vi "create.vi"(8 "error in (no error)":errorcluster, 10 "SubnetSettings":T1, 11 "SubnetFactory in":refnum<class "SubnetFactory.lvclass">) -> (0 "error out":errorcluster, 2 "Subnet":refnum<class "Subnet.lvclass">, 3 "SubnetFactory out":refnum<class "SubnetFactory.lvclass">)   [LabVIEW 2016, in "SubnetFactory.lvclass"]
uses:
  SubnetFactory.lvclass
  Subnet/DataTypes/SubnetSettings.ctl
  Common_RT_Modbus/IModbusFactory/IModbusFactory.lvclass
  Common_RT_HPILC/DataTypes/HPSettings.ctl
  Common_RT_ILC/DataTypes/ILCSettings.ctl
  Common_RT_MTILC/DataTypes/MTSettings.ctl
  Common_RT_MDILC/DataTypes/MDSettings.ctl
  Common_RT_MIILC/DataTypes/MISettings.ctl
  Subnet/Subnet.lvclass
  Common_RT_HPILC/HPILCFactory/HPILCFactory.lvclass
  Subnet/DataTypes/SubnetConstants.ctl
  Common_RT_Modbus/IModbus/IModbus.lvclass
  Common_RT_HPILC/HPILC/HPILC.lvclass
  Subnet/DataTypes/ILCIndexData.ctl
  Subnet/DataTypes/ILCTypes.ctl
  Common_RT_MTILC/MTILC/MTILC.lvclass
  Common_RT_MDILC/MDILC/MDILC.lvclass
  Common_RT_MIILC/MIILC/MIILC.lvclass
  Subnet/DataTypes/SubnetData.ctl
  Subnet/DataTypes/SubnetCommand.ctl
  Subnet/DataTypes/SubnetTelemetry.ctl
  Common_RT_MTILC/MTILCFactory/MTILCFactory.lvclass
  Common_RT_MDILC/MDILCFactory/MDILCFactory.lvclass
  Common_RT_MIILC/MIILCFactory/MIILCFactory.lvclass
  Common_RT_ILC/DataTypes/ILCTimings.ctl
  Common_RT_HPILC/DataTypes/HPTimings.ctl
  Common_RT_MTILC/DataTypes/MTTimings.ctl
  Common_RT_MDILC/DataTypes/MDTimings.ctl
  Common_RT_MIILC/DataTypes/MITimings.ctl
  Subnet/Subnet.lvclass/Subnet.ctl
  Common_RT_ILC/RTILC.lvlib
  Common_RT_HPILC/RTHPILC.lvlib
  Common_RT_MTILC/RTMTILC.lvlib
  Common_RT_MDILC/RTMDILC.lvlib
  Common_RT_MIILC/RTMIILC.lvlib
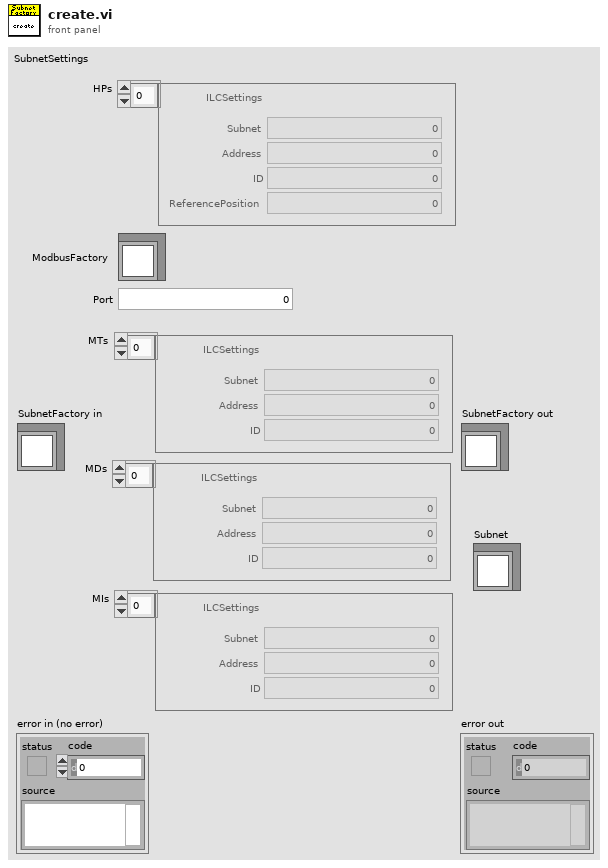
[diagram p1: front panel]
types:
  T1 = typedef "SubnetSettings.ctl" = cluster{"HPs":T2[], "ModbusFactory":refnum<class "IModbusFactory.lvclass">, "Port":i32, "MTs":T4[], "MDs":T5[], "MIs":T6[]}
  T2 = typedef "RTHPILC.lvlib/HPSettings.ctl" = cluster{"ILCSettings":T3, "ID":i16, "ReferencePosition":i32}
  T3 = typedef "RTILC.lvlib/ILCSettings.ctl" = cluster{"Subnet":u8, "Address":u8}
  T4 = typedef "RTMTILC.lvlib/MTSettings.ctl" = cluster{"ILCSettings":T3, "ID":i16}
  T5 = typedef "RTMDILC.lvlib/MDSettings.ctl" = cluster{"ILCSettings":T3, "ID":i16}
  T6 = typedef "RTMIILC.lvlib/MISettings.ctl" = cluster{"ILCSettings":T3, "ID":i16}
  T7 = typedef "RTMIILC.lvlib/MITimings.ctl" = cluster{"Inclination":u32}
  T8 = typedef "RTMDILC.lvlib/MDTimings.ctl" = cluster{"Displacement":u32}
  T9 = typedef "RTMTILC.lvlib/MTTimings.ctl" = cluster{"Temperature":u32}
  T10 = typedef "RTHPILC.lvlib/HPTimings.ctl" = cluster{"BroadcastStepMotor":u32, "ForceAndStatus":u32, "FreezeSensorValues":u32, "StepMotor":u32}
  T11 = typedef "RTILC.lvlib/ILCTimings.ctl" = cluster{"ADCOffsetSensitivity":u32, "ADCScanRate":u32, "ILCMode":u32, "ReadCalibration":u32, "ReportServerID":u32, "ReportServerStatus":u32, "Reset":u32, "SetTemporaryAddress":u32}
  T12 = typedef "SubnetData.ctl" = cluster{"SubnetConstants":T13, "SubnetCommand":T16, "SubnetTelemetry":T17}
  T13 = typedef "SubnetConstants.ctl" = cluster{"Modbus":refnum<class "IModbus.lvclass">, "HPs":refnum<class "HPILC.lvclass">[], "AddressToActuator":T14[], "MTs":refnum<class "MTILC.lvclass">[], "MDs":refnum<class "MDILC.lvclass">[], "MIs":refnum<class "MIILC.lvclass">[]}
  T14 = typedef "ILCIndexData.ctl" = cluster{"ILCTypes":T15, "Index":i32}
  T15 = typedef "ILCTypes.ctl" = enum16{"Undefined", "SAA", "DAA", "HP", "MT", "MD", "MI"}
  T16 = typedef "SubnetCommand.ctl" = cluster{"BroadcastCounter":u8}
  T17 = typedef "SubnetTelemetry.ctl" = cluster{"BytesTransmitted":u32, "FramesTransmitted":u32, "BytesReceived":u32, "FramesReceived":u32, "TxInternalFIFOOverflow":bool, "InvalidInstruction":bool, "WaitForRxFrameTimeout":bool, "StartBitError":bool, "StopBitError":bool, "RxDataFIFOOverflow":bool}
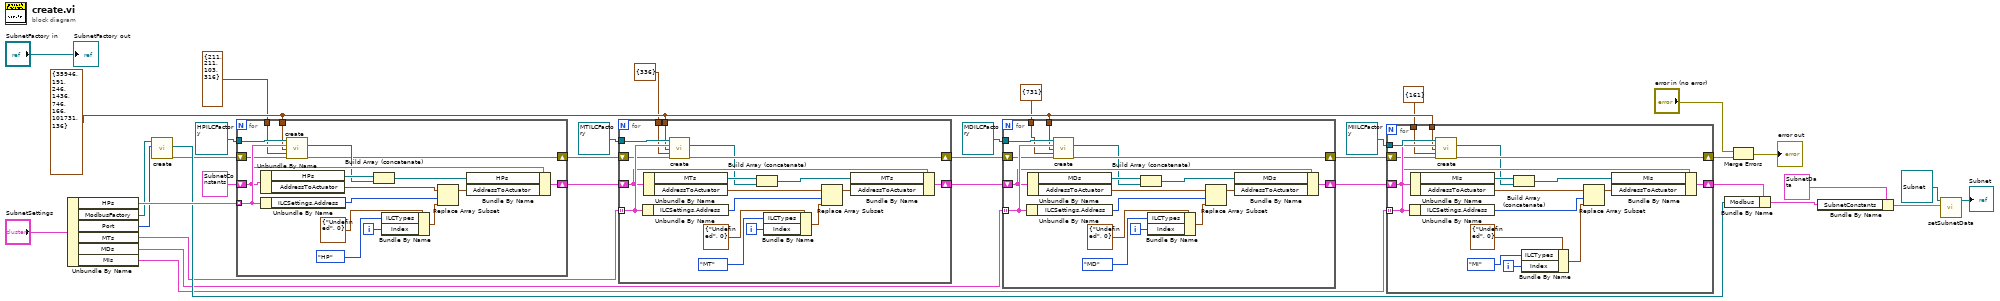
[diagram p0: block diagram]
diagram:
  w5 = T11 {"ADCOffsetSensitivity"=35946, "ADCScanRate"=191, "ILCMode"=246, "ReadCalibration"=1436, "ReportServerID"=746, "ReportServerStatus"=166, "Reset"=101731, "SetTemporaryAddress"=136} ("ILCTimings")
  n1 = Unbundle By Name("SubnetSettings") -> ("HPs"=w33:T2[], "ModbusFactory"=w24:refnum<class "IModbusFactory.lvclass">, "Port"=w23:i32, "MTs"=w19:T4[], "MDs"=w13:T5[], "MIs"=w9:T6[])
  n2 = call-dynamic "create.vi"("Port"=w23, "IModbusFactory in"=w24) -> ("error out"=w21:errorcluster, "IModbus"=w22:refnum<class "IModbus.lvclass">)  [unwired: 7 in, 1 out]
  n3 = for {
    tunnel: w33 -> [w52] mode=indexing
    tunnel: refnum<class "HPILCFactory.lvclass"> refnum ("RTHPILC.lvlib:HPILCFactory.lvclass") -> [w53]
    shift-right: [w43] -> w18
    shift-left: T13 {"Modbus"=refnum, "HPs"=[], "AddressToActuator"=[{"ILCTypes"=enum."Undefined", "Index"=0}, {"ILCTypes"=enum."Undefined", "Index"=0}, {"ILCTypes"=enum."Undefined", "Index"=0}, {"ILCTypes"=enum."Undefined", "Index"=0}, {"ILCTypes"=enum."Undefined", "Index"=0}, {"ILCTypes"=enum."Undefined", "Index"=0}, {"ILCTypes"=enum."Undefined", "Index"=0}, {"ILCTypes"=enum."Undefined", "Index"=0}, {"ILCTypes"=enum."Undefined", "Index"=0}, {"ILCTypes"=enum."Undefined", "Index"=0}, {"ILCTypes"=enum."Undefined", "Index"=0}, {"ILCTypes"=enum."Undefined", "Index"=0}, {"ILCTypes"=enum."Undefined", "Index"=0}, {"ILCTypes"=enum."Undefined", "Index"=0}, {"ILCTypes"=enum."Undefined", "Index"=0}, {"ILCTypes"=enum."Undefined", "Index"=0}, {"ILCTypes"=enum."Undefined", "Index"=0}, {"ILCTypes"=enum."Undefined", "Index"=0}, {"ILCTypes"=enum."Undefined", "Index"=0}, {"ILCTypes"=enum."Undefined", "Index"=0}, {"ILCTypes"=enum."Undefined", "Index"=0}, {"ILCTypes"=enum."Undefined", "Index"=0}, {"ILCTypes"=enum."Undefined", "Index"=0}, {"ILCTypes"=enum."Undefined", "Index"=0}, {"ILCTypes"=enum."Undefined", "Index"=0}, {"ILCTypes"=enum."Undefined", "Index"=0}, {"ILCTypes"=enum."Undefined", "Index"=0}, {"ILCTypes"=enum."Undefined", "Index"=0}, {"ILCTypes"=enum."Undefined", "Index"=0}, {"ILCTypes"=enum."Undefined", "Index"=0}, {"ILCTypes"=enum."Undefined", "Index"=0}, {"ILCTypes"=enum."Undefined", "Index"=0}, {"ILCTypes"=enum."Undefined", "Index"=0}, {"ILCTypes"=enum."Undefined", "Index"=0}, {"ILCTypes"=enum."Undefined", "Index"=0}, {"ILCTypes"=enum."Undefined", "Index"=0}, {"ILCTypes"=enum."Undefined", "Index"=0}, {"ILCTypes"=enum."Undefined", "Index"=0}, {"ILCTypes"=enum."Undefined", "Index"=0}, {"ILCTypes"=enum."Undefined", "Index"=0}, {"ILCTypes"=enum."Undefined", "Index"=0}, {"ILCTypes"=enum."Undefined", "Index"=0}, {"ILCTypes"=enum."Undefined", "Index"=0}, {"ILCTypes"=enum."Undefined", "Index"=0}, {"ILCTypes"=enum."Undefined", "Index"=0}, {"ILCTypes"=enum."Undefined", "Index"=0}, {"ILCTypes"=enum."Undefined", "Index"=0}, {"ILCTypes"=enum."Undefined", "Index"=0}, {"ILCTypes"=enum."Undefined", "Index"=0}, {"ILCTypes"=enum."Undefined", "Index"=0}, {"ILCTypes"=enum."Undefined", "Index"=0}, {"ILCTypes"=enum."Undefined", "Index"=0}, {"ILCTypes"=enum."Undefined", "Index"=0}, {"ILCTypes"=enum."Undefined", "Index"=0}, {"ILCTypes"=enum."Undefined", "Index"=0}, {"ILCTypes"=enum."Undefined", "Index"=0}, {"ILCTypes"=enum."Undefined", "Index"=0}, {"ILCTypes"=enum."Undefined", "Index"=0}, {"ILCTypes"=enum."Undefined", "Index"=0}, {"ILCTypes"=enum."Undefined", "Index"=0}, {"ILCTypes"=enum."Undefined", "Index"=0}, {"ILCTypes"=enum."Undefined", "Index"=0}, {"ILCTypes"=enum."Undefined", "Index"=0}, {"ILCTypes"=enum."Undefined", "Index"=0}, {"ILCTypes"=enum."Undefined", "Index"=0}, {"ILCTypes"=enum."Undefined", "Index"=0}, {"ILCTypes"=enum."Undefined", "Index"=0}, {"ILCTypes"=enum."Undefined", "Index"=0}, {"ILCTypes"=enum."Undefined", "Index"=0}, {"ILCTypes"=enum."Undefined", "Index"=0}, {"ILCTypes"=enum."Undefined", "Index"=0}, {"ILCTypes"=enum."Undefined", "Index"=0}, {"ILCTypes"=enum."Undefined", "Index"=0}, {"ILCTypes"=enum."Undefined", "Index"=0}, {"ILCTypes"=enum."Undefined", "Index"=0}, {"ILCTypes"=enum."Undefined", "Index"=0}, {"ILCTypes"=enum."Undefined", "Index"=0}, {"ILCTypes"=enum."Undefined", "Index"=0}, {"ILCTypes"=enum."Undefined", "Index"=0}, {"ILCTypes"=enum."Undefined", "Index"=0}, {"ILCTypes"=enum."Undefined", "Index"=0}, {"ILCTypes"=enum."Undefined", "Index"=0}, {"ILCTypes"=enum."Undefined", "Index"=0}, {"ILCTypes"=enum."Undefined", "Index"=0}, {"ILCTypes"=enum."Undefined", "Index"=0}, {"ILCTypes"=enum."Undefined", "Index"=0}, {"ILCTypes"=enum."Undefined", "Index"=0}, {"ILCTypes"=enum."Undefined", "Index"=0}, {"ILCTypes"=enum."Undefined", "Index"=0}, {"ILCTypes"=enum."Undefined", "Index"=0}, {"ILCTypes"=enum."Undefined", "Index"=0}, {"ILCTypes"=enum."Undefined", "Index"=0}, {"ILCTypes"=enum."Undefined", "Index"=0}, {"ILCTypes"=enum."Undefined", "Index"=0}, {"ILCTypes"=enum."Undefined", "Index"=0}, {"ILCTypes"=enum."Undefined", "Index"=0}, {"ILCTypes"=enum."Undefined", "Index"=0}, {"ILCTypes"=enum."Undefined", "Index"=0}, {"ILCTypes"=enum."Undefined", "Index"=0}, {"ILCTypes"=enum."Undefined", "Index"=0}, {"ILCTypes"=enum."Undefined", "Index"=0}, {"ILCTypes"=enum."Undefined", "Index"=0}, {"ILCTypes"=enum."Undefined", "Index"=0}, {"ILCTypes"=enum."Undefined", "Index"=0}, {"ILCTypes"=enum."Undefined", "Index"=0}, {"ILCTypes"=enum."Undefined", "Index"=0}, {"ILCTypes"=enum."Undefined", "Index"=0}, {"ILCTypes"=enum."Undefined", "Index"=0}, {"ILCTypes"=enum."Undefined", "Index"=0}, {"ILCTypes"=enum."Undefined", "Index"=0}, {"ILCTypes"=enum."Undefined", "Index"=0}, {"ILCTypes"=enum."Undefined", "Index"=0}, {"ILCTypes"=enum."Undefined", "Index"=0}, {"ILCTypes"=enum."Undefined", "Index"=0}, {"ILCTypes"=enum."Undefined", "Index"=0}, {"ILCTypes"=enum."Undefined", "Index"=0}, {"ILCTypes"=enum."Undefined", "Index"=0}, {"ILCTypes"=enum."Undefined", "Index"=0}, {"ILCTypes"=enum."Undefined", "Index"=0}, {"ILCTypes"=enum."Undefined", "Index"=0}, {"ILCTypes"=enum."Undefined", "Index"=0}, {"ILCTypes"=enum."Undefined", "Index"=0}, {"ILCTypes"=enum."Undefined", "Index"=0}, {"ILCTypes"=enum."Undefined", "Index"=0}, {"ILCTypes"=enum."Undefined", "Index"=0}, {"ILCTypes"=enum."Undefined", "Index"=0}, {"ILCTypes"=enum."Undefined", "Index"=0}, {"ILCTypes"=enum."Undefined", "Index"=0}, {"ILCTypes"=enum."Undefined", "Index"=0}, {"ILCTypes"=enum."Undefined", "Index"=0}, {"ILCTypes"=enum."Undefined", "Index"=0}, {"ILCTypes"=enum."Undefined", "Index"=0}, {"ILCTypes"=enum."Undefined", "Index"=0}, {"ILCTypes"=enum."Undefined", "Index"=0}, {"ILCTypes"=enum."Undefined", "Index"=0}, {"ILCTypes"=enum."Undefined", "Index"=0}, {"ILCTypes"=enum."Undefined", "Index"=0}, {"ILCTypes"=enum."Undefined", "Index"=0}, {"ILCTypes"=enum."Undefined", "Index"=0}, {"ILCTypes"=enum."Undefined", "Index"=0}, {"ILCTypes"=enum."Undefined", "Index"=0}, {"ILCTypes"=enum."Undefined", "Index"=0}, {"ILCTypes"=enum."Undefined", "Index"=0}, {"ILCTypes"=enum."Undefined", "Index"=0}, {"ILCTypes"=enum."Undefined", "Index"=0}, {"ILCTypes"=enum."Undefined", "Index"=0}, {"ILCTypes"=enum."Undefined", "Index"=0}, {"ILCTypes"=enum."Undefined", "Index"=0}, {"ILCTypes"=enum."Undefined", "Index"=0}, {"ILCTypes"=enum."Undefined", "Index"=0}, {"ILCTypes"=enum."Undefined", "Index"=0}, {"ILCTypes"=enum."Undefined", "Index"=0}, {"ILCTypes"=enum."Undefined", "Index"=0}, {"ILCTypes"=enum."Undefined", "Index"=0}, {"ILCTypes"=enum."Undefined", "Index"=0}, {"ILCTypes"=enum."Undefined", "Index"=0}, {"ILCTypes"=enum."Undefined", "Index"=0}, {"ILCTypes"=enum."Undefined", "Index"=0}, {"ILCTypes"=enum."Undefined", "Index"=0}, {"ILCTypes"=enum."Undefined", "Index"=0}, {"ILCTypes"=enum."Undefined", "Index"=0}, {"ILCTypes"=enum."Undefined", "Index"=0}, {"ILCTypes"=enum."Undefined", "Index"=0}, {"ILCTypes"=enum."Undefined", "Index"=0}, {"ILCTypes"=enum."Undefined", "Index"=0}, {"ILCTypes"=enum."Undefined", "Index"=0}, {"ILCTypes"=enum."Undefined", "Index"=0}, {"ILCTypes"=enum."Undefined", "Index"=0}, {"ILCTypes"=enum."Undefined", "Index"=0}, {"ILCTypes"=enum."Undefined", "Index"=0}, {"ILCTypes"=enum."Undefined", "Index"=0}, {"ILCTypes"=enum."Undefined", "Index"=0}, {"ILCTypes"=enum."Undefined", "Index"=0}, {"ILCTypes"=enum."Undefined", "Index"=0}, {"ILCTypes"=enum."Undefined", "Index"=0}, {"ILCTypes"=enum."Undefined", "Index"=0}, {"ILCTypes"=enum."Undefined", "Index"=0}, {"ILCTypes"=enum."Undefined", "Index"=0}, {"ILCTypes"=enum."Undefined", "Index"=0}, {"ILCTypes"=enum."Undefined", "Index"=0}, {"ILCTypes"=enum."Undefined", "Index"=0}, {"ILCTypes"=enum."Undefined", "Index"=0}, {"ILCTypes"=enum."Undefined", "Index"=0}, {"ILCTypes"=enum."Undefined", "Index"=0}, {"ILCTypes"=enum."Undefined", "Index"=0}, {"ILCTypes"=enum."Undefined", "Index"=0}, {"ILCTypes"=enum."Undefined", "Index"=0}, {"ILCTypes"=enum."Undefined", "Index"=0}, {"ILCTypes"=enum."Undefined", "Index"=0}, {"ILCTypes"=enum."Undefined", "Index"=0}, {"ILCTypes"=enum."Undefined", "Index"=0}, {"ILCTypes"=enum."Undefined", "Index"=0}, {"ILCTypes"=enum."Undefined", "Index"=0}, {"ILCTypes"=enum."Undefined", "Index"=0}, {"ILCTypes"=enum."Undefined", "Index"=0}, {"ILCTypes"=enum."Undefined", "Index"=0}, {"ILCTypes"=enum."Undefined", "Index"=0}, {"ILCTypes"=enum."Undefined", "Index"=0}, {"ILCTypes"=enum."Undefined", "Index"=0}, {"ILCTypes"=enum."Undefined", "Index"=0}, {"ILCTypes"=enum."Undefined", "Index"=0}, {"ILCTypes"=enum."Undefined", "Index"=0}, {"ILCTypes"=enum."Undefined", "Index"=0}, {"ILCTypes"=enum."Undefined", "Index"=0}, {"ILCTypes"=enum."Undefined", "Index"=0}, {"ILCTypes"=enum."Undefined", "Index"=0}, {"ILCTypes"=enum."Undefined", "Index"=0}, {"ILCTypes"=enum."Undefined", "Index"=0}, {"ILCTypes"=enum."Undefined", "Index"=0}, {"ILCTypes"=enum."Undefined", "Index"=0}, {"ILCTypes"=enum."Undefined", "Index"=0}, {"ILCTypes"=enum."Undefined", "Index"=0}, {"ILCTypes"=enum."Undefined", "Index"=0}, {"ILCTypes"=enum."Undefined", "Index"=0}, {"ILCTypes"=enum."Undefined", "Index"=0}, {"ILCTypes"=enum."Undefined", "Index"=0}, {"ILCTypes"=enum."Undefined", "Index"=0}, {"ILCTypes"=enum."Undefined", "Index"=0}, {"ILCTypes"=enum."Undefined", "Index"=0}, {"ILCTypes"=enum."Undefined", "Index"=0}, {"ILCTypes"=enum."Undefined", "Index"=0}, {"ILCTypes"=enum."Undefined", "Index"=0}, {"ILCTypes"=enum."Undefined", "Index"=0}, {"ILCTypes"=enum."Undefined", "Index"=0}, {"ILCTypes"=enum."Undefined", "Index"=0}, {"ILCTypes"=enum."Undefined", "Index"=0}, {"ILCTypes"=enum."Undefined", "Index"=0}, {"ILCTypes"=enum."Undefined", "Index"=0}, {"ILCTypes"=enum."Undefined", "Index"=0}, {"ILCTypes"=enum."Undefined", "Index"=0}, {"ILCTypes"=enum."Undefined", "Index"=0}, {"ILCTypes"=enum."Undefined", "Index"=0}, {"ILCTypes"=enum."Undefined", "Index"=0}, {"ILCTypes"=enum."Undefined", "Index"=0}, {"ILCTypes"=enum."Undefined", "Index"=0}, {"ILCTypes"=enum."Undefined", "Index"=0}, {"ILCTypes"=enum."Undefined", "Index"=0}, {"ILCTypes"=enum."Undefined", "Index"=0}, {"ILCTypes"=enum."Undefined", "Index"=0}, {"ILCTypes"=enum."Undefined", "Index"=0}, {"ILCTypes"=enum."Undefined", "Index"=0}, {"ILCTypes"=enum."Undefined", "Index"=0}, {"ILCTypes"=enum."Undefined", "Index"=0}, {"ILCTypes"=enum."Undefined", "Index"=0}, {"ILCTypes"=enum."Undefined", "Index"=0}, {"ILCTypes"=enum."Undefined", "Index"=0}, {"ILCTypes"=enum."Undefined", "Index"=0}, {"ILCTypes"=enum."Undefined", "Index"=0}, {"ILCTypes"=enum."Undefined", "Index"=0}, {"ILCTypes"=enum."Undefined", "Index"=0}, {"ILCTypes"=enum."Undefined", "Index"=0}, {"ILCTypes"=enum."Undefined", "Index"=0}, {"ILCTypes"=enum."Undefined", "Index"=0}, {"ILCTypes"=enum."Undefined", "Index"=0}, {"ILCTypes"=enum."Undefined", "Index"=0}, {"ILCTypes"=enum."Undefined", "Index"=0}], "MTs"=[], "MDs"=[], "MIs"=[]} ("SubnetConstants") -> [w45]
    shift-right: [w38] -> w17
    shift-left: w21 -> [w42]
    tunnel: w5 -> [w37]
    tunnel: T10 {"BroadcastStepMotor"=211, "ForceAndStatus"=211, "FreezeSensorValues"=103, "StepMotor"=316} ("HPTimings") -> [w36]
    i -> [w48]
    n4 = Unbundle By Name(w52) -> ("ILCSettings.Address"=w51:u8)
    n5 = Unbundle By Name(w45) -> ("HPs"=w41:refnum<class "HPILC.lvclass">[], "AddressToActuator"=w50:T14[])
    n6 = call "create.vi"("HPILCFactory in"=w53, "HPSettings"=w52, "ILCTimings"=w37, "HPTimings"=w36, "error in (no error)"=w42) -> ("HPILC"=w40:refnum<class "HPILC.lvclass">, "error out"=w38:errorcluster)  [unwired: 8 in, 1 out]
    n7 = Build Array (concatenate)(w41, w40) -> (w39:refnum<class "HPILC.lvclass">[])
    n8 = Bundle By Name(cluster=T14 {"ILCTypes"=enum."Undefined", "Index"=0} ("new element/subarray"), "ILCTypes"=ILCTypes."HP", "Index"=w48) -> (w46:T14)
    n9 = Replace Array Subset(array=w50, new element=w46, index=w51) -> (w44:T14[])
    n10 = Bundle By Name(cluster=w45, "HPs"=w39, "AddressToActuator"=w44) -> (w43:T13)
  }
  n11 = for {
    tunnel: w19 -> [w70] mode=indexing
    tunnel: refnum<class "MTILCFactory.lvclass"> refnum ("RTMTILC.lvlib:MTILCFactory.lvclass") -> [w71]
    shift-right: [w61] -> w15
    shift-left: w18 -> [w63]
    shift-right: [w60] -> w16
    shift-left: w17 -> [w59]
    tunnel: w5 -> [w55]
    tunnel: T9 {"Temperature"=336} ("MTTimings") -> [w54]
    i -> [w66]
    n12 = Unbundle By Name(w70) -> ("ILCSettings.Address"=w69:u8)
    n13 = Unbundle By Name(w63) -> ("MTs"=w58:refnum<class "MTILC.lvclass">[], "AddressToActuator"=w68:T14[])
    n14 = call "create.vi"("MTILCFactory in"=w71, "MTSettings"=w70, "ILCTimings"=w55, "MTTimings"=w54, "error in (no error)"=w59) -> ("MTILC"=w57:refnum<class "MTILC.lvclass">, "error out"=w60:errorcluster)  [unwired: 8 in, 1 out]
    n15 = Build Array (concatenate)(w58, w57) -> (w56:refnum<class "MTILC.lvclass">[])
    n16 = Bundle By Name(cluster=T14 {"ILCTypes"=enum."Undefined", "Index"=0} ("new element/subarray"), "ILCTypes"=ILCTypes."MT", "Index"=w66) -> (w64:T14)
    n17 = Replace Array Subset(array=w68, new element=w64, index=w69) -> (w62:T14[])
    n18 = Bundle By Name(cluster=w63, "MTs"=w56, "AddressToActuator"=w62) -> (w61:T13)
  }
  n19 = for {
    tunnel: w13 -> [w88] mode=indexing
    tunnel: refnum<class "MDILCFactory.lvclass"> refnum ("RTMDILC.lvlib:MDILCFactory.lvclass") -> [w89]
    shift-right: [w79] -> w10
    shift-left: w15 -> [w81]
    shift-right: [w78] -> w11
    shift-left: w16 -> [w77]
    tunnel: w5 -> [w73]
    tunnel: T8 {"Displacement"=731} ("MDTimings") -> [w72]
    i -> [w84]
    n20 = Unbundle By Name(w88) -> ("ILCSettings.Address"=w87:u8)
    n21 = Unbundle By Name(w81) -> ("MDs"=w76:refnum<class "MDILC.lvclass">[], "AddressToActuator"=w86:T14[])
    n22 = call "create.vi"("MDILCFactory in"=w89, "MDSettings"=w88, "ILCTimings"=w73, "MDTimings"=w72, "error in (no error)"=w77) -> ("MDILC"=w75:refnum<class "MDILC.lvclass">, "error out"=w78:errorcluster)  [unwired: 8 in, 1 out]
    n23 = Build Array (concatenate)(w76, w75) -> (w74:refnum<class "MDILC.lvclass">[])
    n24 = Bundle By Name(cluster=T14 {"ILCTypes"=enum."Undefined", "Index"=0} ("new element/subarray"), "ILCTypes"=ILCTypes."MD", "Index"=w84) -> (w82:T14)
    n25 = Replace Array Subset(array=w86, new element=w82, index=w87) -> (w80:T14[])
    n26 = Bundle By Name(cluster=w81, "MDs"=w74, "AddressToActuator"=w80) -> (w79:T13)
  }
  n27 = for {
    tunnel: w9 -> [w106] mode=indexing
    tunnel: refnum<class "MIILCFactory.lvclass"> refnum ("RTMIILC.lvlib:MIILCFactory.lvclass") -> [w107]
    shift-right: [w97] -> w7
    shift-left: w10 -> [w99]
    shift-right: [w96] -> w8
    shift-left: w11 -> [w95]
    tunnel: w5 -> [w91]
    tunnel: T7 {"Inclination"=161} ("MITimings") -> [w90]
    i -> [w102]
    n28 = Unbundle By Name(w106) -> ("ILCSettings.Address"=w105:u8)
    n29 = Unbundle By Name(w99) -> ("MIs"=w94:refnum<class "MIILC.lvclass">[], "AddressToActuator"=w104:T14[])
    n30 = call "create.vi"("MIILCFactory in"=w107, "MISettings"=w106, "ILCTimings"=w91, "MITimings"=w90, "error in (no error)"=w95) -> ("MIILC"=w93:refnum<class "MIILC.lvclass">, "error out"=w96:errorcluster)  [unwired: 8 in, 1 out]
    n31 = Build Array (concatenate)(w94, w93) -> (w92:refnum<class "MIILC.lvclass">[])
    n32 = Bundle By Name(cluster=T14 {"ILCTypes"=enum."Undefined", "Index"=0} ("new element/subarray"), "ILCTypes"=ILCTypes."MI", "Index"=w102) -> (w100:T14)
    n33 = Replace Array Subset(array=w104, new element=w100, index=w105) -> (w98:T14[])
    n34 = Bundle By Name(cluster=w99, "MIs"=w92, "AddressToActuator"=w98) -> (w97:T13)
  }
  n35 = Bundle By Name(cluster=w7, "Modbus"=w22) -> (w6:T13)
  n36 = Merge Errors("error in (no error)", w8) -> (→"error out":errorcluster)
  n37 = Bundle By Name(cluster=T12 {"SubnetConstants"={"Modbus"=refnum, "HPs"=[], "AddressToActuator"=[{"ILCTypes"=enum."Undefined", "Index"=0}, {"ILCTypes"=enum."Undefined", "Index"=0}, {"ILCTypes"=enum."Undefined", "Index"=0}, {"ILCTypes"=enum."Undefined", "Index"=0}, {"ILCTypes"=enum."Undefined", "Index"=0}, {"ILCTypes"=enum."Undefined", "Index"=0}, {"ILCTypes"=enum."Undefined", "Index"=0}, {"ILCTypes"=enum."Undefined", "Index"=0}, {"ILCTypes"=enum."Undefined", "Index"=0}, {"ILCTypes"=enum."Undefined", "Index"=0}, {"ILCTypes"=enum."Undefined", "Index"=0}, {"ILCTypes"=enum."Undefined", "Index"=0}, {"ILCTypes"=enum."Undefined", "Index"=0}, {"ILCTypes"=enum."Undefined", "Index"=0}, {"ILCTypes"=enum."Undefined", "Index"=0}, {"ILCTypes"=enum."Undefined", "Index"=0}, {"ILCTypes"=enum."Undefined", "Index"=0}, {"ILCTypes"=enum."Undefined", "Index"=0}, {"ILCTypes"=enum."Undefined", "Index"=0}, {"ILCTypes"=enum."Undefined", "Index"=0}, {"ILCTypes"=enum."Undefined", "Index"=0}, {"ILCTypes"=enum."Undefined", "Index"=0}, {"ILCTypes"=enum."Undefined", "Index"=0}, {"ILCTypes"=enum."Undefined", "Index"=0}, {"ILCTypes"=enum."Undefined", "Index"=0}, {"ILCTypes"=enum."Undefined", "Index"=0}, {"ILCTypes"=enum."Undefined", "Index"=0}, {"ILCTypes"=enum."Undefined", "Index"=0}, {"ILCTypes"=enum."Undefined", "Index"=0}, {"ILCTypes"=enum."Undefined", "Index"=0}, {"ILCTypes"=enum."Undefined", "Index"=0}, {"ILCTypes"=enum."Undefined", "Index"=0}, {"ILCTypes"=enum."Undefined", "Index"=0}, {"ILCTypes"=enum."Undefined", "Index"=0}, {"ILCTypes"=enum."Undefined", "Index"=0}, {"ILCTypes"=enum."Undefined", "Index"=0}, {"ILCTypes"=enum."Undefined", "Index"=0}, {"ILCTypes"=enum."Undefined", "Index"=0}, {"ILCTypes"=enum."Undefined", "Index"=0}, {"ILCTypes"=enum."Undefined", "Index"=0}, {"ILCTypes"=enum."Undefined", "Index"=0}, {"ILCTypes"=enum."Undefined", "Index"=0}, {"ILCTypes"=enum."Undefined", "Index"=0}, {"ILCTypes"=enum."Undefined", "Index"=0}, {"ILCTypes"=enum."Undefined", "Index"=0}, {"ILCTypes"=enum."Undefined", "Index"=0}, {"ILCTypes"=enum."Undefined", "Index"=0}, {"ILCTypes"=enum."Undefined", "Index"=0}, {"ILCTypes"=enum."Undefined", "Index"=0}, {"ILCTypes"=enum."Undefined", "Index"=0}, {"ILCTypes"=enum."Undefined", "Index"=0}, {"ILCTypes"=enum."Undefined", "Index"=0}, {"ILCTypes"=enum."Undefined", "Index"=0}, {"ILCTypes"=enum."Undefined", "Index"=0}, {"ILCTypes"=enum."Undefined", "Index"=0}, {"ILCTypes"=enum."Undefined", "Index"=0}, {"ILCTypes"=enum."Undefined", "Index"=0}, {"ILCTypes"=enum."Undefined", "Index"=0}, {"ILCTypes"=enum."Undefined", "Index"=0}, {"ILCTypes"=enum."Undefined", "Index"=0}, {"ILCTypes"=enum."Undefined", "Index"=0}, {"ILCTypes"=enum."Undefined", "Index"=0}, {"ILCTypes"=enum."Undefined", "Index"=0}, {"ILCTypes"=enum."Undefined", "Index"=0}, {"ILCTypes"=enum."Undefined", "Index"=0}, {"ILCTypes"=enum."Undefined", "Index"=0}, {"ILCTypes"=enum."Undefined", "Index"=0}, {"ILCTypes"=enum."Undefined", "Index"=0}, {"ILCTypes"=enum."Undefined", "Index"=0}, {"ILCTypes"=enum."Undefined", "Index"=0}, {"ILCTypes"=enum."Undefined", "Index"=0}, {"ILCTypes"=enum."Undefined", "Index"=0}, {"ILCTypes"=enum."Undefined", "Index"=0}, {"ILCTypes"=enum."Undefined", "Index"=0}, {"ILCTypes"=enum."Undefined", "Index"=0}, {"ILCTypes"=enum."Undefined", "Index"=0}, {"ILCTypes"=enum."Undefined", "Index"=0}, {"ILCTypes"=enum."Undefined", "Index"=0}, {"ILCTypes"=enum."Undefined", "Index"=0}, {"ILCTypes"=enum."Undefined", "Index"=0}, {"ILCTypes"=enum."Undefined", "Index"=0}, {"ILCTypes"=enum."Undefined", "Index"=0}, {"ILCTypes"=enum."Undefined", "Index"=0}, {"ILCTypes"=enum."Undefined", "Index"=0}, {"ILCTypes"=enum."Undefined", "Index"=0}, {"ILCTypes"=enum."Undefined", "Index"=0}, {"ILCTypes"=enum."Undefined", "Index"=0}, {"ILCTypes"=enum."Undefined", "Index"=0}, {"ILCTypes"=enum."Undefined", "Index"=0}, {"ILCTypes"=enum."Undefined", "Index"=0}, {"ILCTypes"=enum."Undefined", "Index"=0}, {"ILCTypes"=enum."Undefined", "Index"=0}, {"ILCTypes"=enum."Undefined", "Index"=0}, {"ILCTypes"=enum."Undefined", "Index"=0}, {"ILCTypes"=enum."Undefined", "Index"=0}, {"ILCTypes"=enum."Undefined", "Index"=0}, {"ILCTypes"=enum."Undefined", "Index"=0}, {"ILCTypes"=enum."Undefined", "Index"=0}, {"ILCTypes"=enum."Undefined", "Index"=0}, {"ILCTypes"=enum."Undefined", "Index"=0}, {"ILCTypes"=enum."Undefined", "Index"=0}, {"ILCTypes"=enum."Undefined", "Index"=0}, {"ILCTypes"=enum."Undefined", "Index"=0}, {"ILCTypes"=enum."Undefined", "Index"=0}, {"ILCTypes"=enum."Undefined", "Index"=0}, {"ILCTypes"=enum."Undefined", "Index"=0}, {"ILCTypes"=enum."Undefined", "Index"=0}, {"ILCTypes"=enum."Undefined", "Index"=0}, {"ILCTypes"=enum."Undefined", "Index"=0}, {"ILCTypes"=enum."Undefined", "Index"=0}, {"ILCTypes"=enum."Undefined", "Index"=0}, {"ILCTypes"=enum."Undefined", "Index"=0}, {"ILCTypes"=enum."Undefined", "Index"=0}, {"ILCTypes"=enum."Undefined", "Index"=0}, {"ILCTypes"=enum."Undefined", "Index"=0}, {"ILCTypes"=enum."Undefined", "Index"=0}, {"ILCTypes"=enum."Undefined", "Index"=0}, {"ILCTypes"=enum."Undefined", "Index"=0}, {"ILCTypes"=enum."Undefined", "Index"=0}, {"ILCTypes"=enum."Undefined", "Index"=0}, {"ILCTypes"=enum."Undefined", "Index"=0}, {"ILCTypes"=enum."Undefined", "Index"=0}, {"ILCTypes"=enum."Undefined", "Index"=0}, {"ILCTypes"=enum."Undefined", "Index"=0}, {"ILCTypes"=enum."Undefined", "Index"=0}, {"ILCTypes"=enum."Undefined", "Index"=0}, {"ILCTypes"=enum."Undefined", "Index"=0}, {"ILCTypes"=enum."Undefined", "Index"=0}, {"ILCTypes"=enum."Undefined", "Index"=0}, {"ILCTypes"=enum."Undefined", "Index"=0}, {"ILCTypes"=enum."Undefined", "Index"=0}, {"ILCTypes"=enum."Undefined", "Index"=0}, {"ILCTypes"=enum."Undefined", "Index"=0}, {"ILCTypes"=enum."Undefined", "Index"=0}, {"ILCTypes"=enum."Undefined", "Index"=0}, {"ILCTypes"=enum."Undefined", "Index"=0}, {"ILCTypes"=enum."Undefined", "Index"=0}, {"ILCTypes"=enum."Undefined", "Index"=0}, {"ILCTypes"=enum."Undefined", "Index"=0}, {"ILCTypes"=enum."Undefined", "Index"=0}, {"ILCTypes"=enum."Undefined", "Index"=0}, {"ILCTypes"=enum."Undefined", "Index"=0}, {"ILCTypes"=enum."Undefined", "Index"=0}, {"ILCTypes"=enum."Undefined", "Index"=0}, {"ILCTypes"=enum."Undefined", "Index"=0}, {"ILCTypes"=enum."Undefined", "Index"=0}, {"ILCTypes"=enum."Undefined", "Index"=0}, {"ILCTypes"=enum."Undefined", "Index"=0}, {"ILCTypes"=enum."Undefined", "Index"=0}, {"ILCTypes"=enum."Undefined", "Index"=0}, {"ILCTypes"=enum."Undefined", "Index"=0}, {"ILCTypes"=enum."Undefined", "Index"=0}, {"ILCTypes"=enum."Undefined", "Index"=0}, {"ILCTypes"=enum."Undefined", "Index"=0}, {"ILCTypes"=enum."Undefined", "Index"=0}, {"ILCTypes"=enum."Undefined", "Index"=0}, {"ILCTypes"=enum."Undefined", "Index"=0}, {"ILCTypes"=enum."Undefined", "Index"=0}, {"ILCTypes"=enum."Undefined", "Index"=0}, {"ILCTypes"=enum."Undefined", "Index"=0}, {"ILCTypes"=enum."Undefined", "Index"=0}, {"ILCTypes"=enum."Undefined", "Index"=0}, {"ILCTypes"=enum."Undefined", "Index"=0}, {"ILCTypes"=enum."Undefined", "Index"=0}, {"ILCTypes"=enum."Undefined", "Index"=0}, {"ILCTypes"=enum."Undefined", "Index"=0}, {"ILCTypes"=enum."Undefined", "Index"=0}, {"ILCTypes"=enum."Undefined", "Index"=0}, {"ILCTypes"=enum."Undefined", "Index"=0}, {"ILCTypes"=enum."Undefined", "Index"=0}, {"ILCTypes"=enum."Undefined", "Index"=0}, {"ILCTypes"=enum."Undefined", "Index"=0}, {"ILCTypes"=enum."Undefined", "Index"=0}, {"ILCTypes"=enum."Undefined", "Index"=0}, {"ILCTypes"=enum."Undefined", "Index"=0}, {"ILCTypes"=enum."Undefined", "Index"=0}, {"ILCTypes"=enum."Undefined", "Index"=0}, {"ILCTypes"=enum."Undefined", "Index"=0}, {"ILCTypes"=enum."Undefined", "Index"=0}, {"ILCTypes"=enum."Undefined", "Index"=0}, {"ILCTypes"=enum."Undefined", "Index"=0}, {"ILCTypes"=enum."Undefined", "Index"=0}, {"ILCTypes"=enum."Undefined", "Index"=0}, {"ILCTypes"=enum."Undefined", "Index"=0}, {"ILCTypes"=enum."Undefined", "Index"=0}, {"ILCTypes"=enum."Undefined", "Index"=0}, {"ILCTypes"=enum."Undefined", "Index"=0}, {"ILCTypes"=enum."Undefined", "Index"=0}, {"ILCTypes"=enum."Undefined", "Index"=0}, {"ILCTypes"=enum."Undefined", "Index"=0}, {"ILCTypes"=enum."Undefined", "Index"=0}, {"ILCTypes"=enum."Undefined", "Index"=0}, {"ILCTypes"=enum."Undefined", "Index"=0}, {"ILCTypes"=enum."Undefined", "Index"=0}, {"ILCTypes"=enum."Undefined", "Index"=0}, {"ILCTypes"=enum."Undefined", "Index"=0}, {"ILCTypes"=enum."Undefined", "Index"=0}, {"ILCTypes"=enum."Undefined", "Index"=0}, {"ILCTypes"=enum."Undefined", "Index"=0}, {"ILCTypes"=enum."Undefined", "Index"=0}, {"ILCTypes"=enum."Undefined", "Index"=0}, {"ILCTypes"=enum."Undefined", "Index"=0}, {"ILCTypes"=enum."Undefined", "Index"=0}, {"ILCTypes"=enum."Undefined", "Index"=0}, {"ILCTypes"=enum."Undefined", "Index"=0}, {"ILCTypes"=enum."Undefined", "Index"=0}, {"ILCTypes"=enum."Undefined", "Index"=0}, {"ILCTypes"=enum."Undefined", "Index"=0}, {"ILCTypes"=enum."Undefined", "Index"=0}, {"ILCTypes"=enum."Undefined", "Index"=0}, {"ILCTypes"=enum."Undefined", "Index"=0}, {"ILCTypes"=enum."Undefined", "Index"=0}, {"ILCTypes"=enum."Undefined", "Index"=0}, {"ILCTypes"=enum."Undefined", "Index"=0}, {"ILCTypes"=enum."Undefined", "Index"=0}, {"ILCTypes"=enum."Undefined", "Index"=0}, {"ILCTypes"=enum."Undefined", "Index"=0}, {"ILCTypes"=enum."Undefined", "Index"=0}, {"ILCTypes"=enum."Undefined", "Index"=0}, {"ILCTypes"=enum."Undefined", "Index"=0}, {"ILCTypes"=enum."Undefined", "Index"=0}, {"ILCTypes"=enum."Undefined", "Index"=0}, {"ILCTypes"=enum."Undefined", "Index"=0}, {"ILCTypes"=enum."Undefined", "Index"=0}, {"ILCTypes"=enum."Undefined", "Index"=0}, {"ILCTypes"=enum."Undefined", "Index"=0}, {"ILCTypes"=enum."Undefined", "Index"=0}, {"ILCTypes"=enum."Undefined", "Index"=0}, {"ILCTypes"=enum."Undefined", "Index"=0}, {"ILCTypes"=enum."Undefined", "Index"=0}, {"ILCTypes"=enum."Undefined", "Index"=0}, {"ILCTypes"=enum."Undefined", "Index"=0}, {"ILCTypes"=enum."Undefined", "Index"=0}, {"ILCTypes"=enum."Undefined", "Index"=0}, {"ILCTypes"=enum."Undefined", "Index"=0}, {"ILCTypes"=enum."Undefined", "Index"=0}, {"ILCTypes"=enum."Undefined", "Index"=0}, {"ILCTypes"=enum."Undefined", "Index"=0}, {"ILCTypes"=enum."Undefined", "Index"=0}, {"ILCTypes"=enum."Undefined", "Index"=0}, {"ILCTypes"=enum."Undefined", "Index"=0}, {"ILCTypes"=enum."Undefined", "Index"=0}, {"ILCTypes"=enum."Undefined", "Index"=0}, {"ILCTypes"=enum."Undefined", "Index"=0}, {"ILCTypes"=enum."Undefined", "Index"=0}, {"ILCTypes"=enum."Undefined", "Index"=0}, {"ILCTypes"=enum."Undefined", "Index"=0}, {"ILCTypes"=enum."Undefined", "Index"=0}, {"ILCTypes"=enum."Undefined", "Index"=0}, {"ILCTypes"=enum."Undefined", "Index"=0}, {"ILCTypes"=enum."Undefined", "Index"=0}, {"ILCTypes"=enum."Undefined", "Index"=0}, {"ILCTypes"=enum."Undefined", "Index"=0}, {"ILCTypes"=enum."Undefined", "Index"=0}, {"ILCTypes"=enum."Undefined", "Index"=0}, {"ILCTypes"=enum."Undefined", "Index"=0}], "MTs"=[], "MDs"=[], "MIs"=[]}, "SubnetCommand"={"BroadcastCounter"=0}, "SubnetTelemetry"={"BytesTransmitted"=0, "FramesTransmitted"=0, "BytesReceived"=0, "FramesReceived"=0, "TxInternalFIFOOverflow"=FALSE, "InvalidInstruction"=FALSE, "WaitForRxFrameTimeout"=FALSE, "StartBitError"=FALSE, "StopBitError"=FALSE, "RxDataFIFOOverflow"=FALSE}} ("SubnetData"), "SubnetConstants"=w6) -> (w27:T12)
  n38 = call "setSubnetData.vi"("SubnetData"=w27, "Subnet in"=refnum<class "Subnet.lvclass"> refnum ("Subnet.lvclass")) -> ("Subnet out"=→"Subnet":refnum<class "Subnet.lvclass">)  [unwired: 9 in]
  "SubnetFactory out" <- "SubnetFactory in"
